vi "Remove - Update Poly Set Map.vi"(8 "error in (no error)":errorcluster, 10 "Data Type to Remove":string[](array[string]), 11 "Poly Set Map in in":T1) -> (0 "error out":errorcluster, 1 "Data Type Library Path":path, 2 "Data Type Directory":path, 3 "Poly Set Map out":T1)   [LabVIEW 2020]
uses:
  _td_map_PolyInstanceInfo.ctl
  _td_cluster_InstanceInfo.ctl
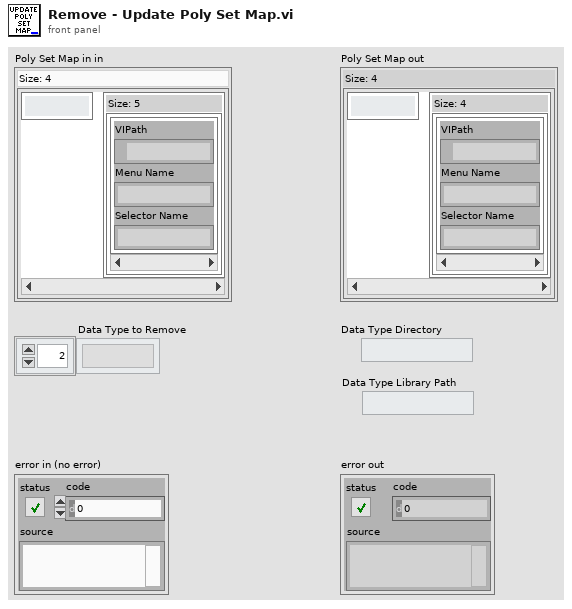
[diagram p1: front panel]
types:
  T1 = typedef "_td_map_PolyInstanceInfo.ctl" = map{string, set{T2}}
  T2 = typedef "_td_cluster_InstanceInfo.ctl" = cluster{"VIPath":path, "Menu Name":string, "Selector Name":string}
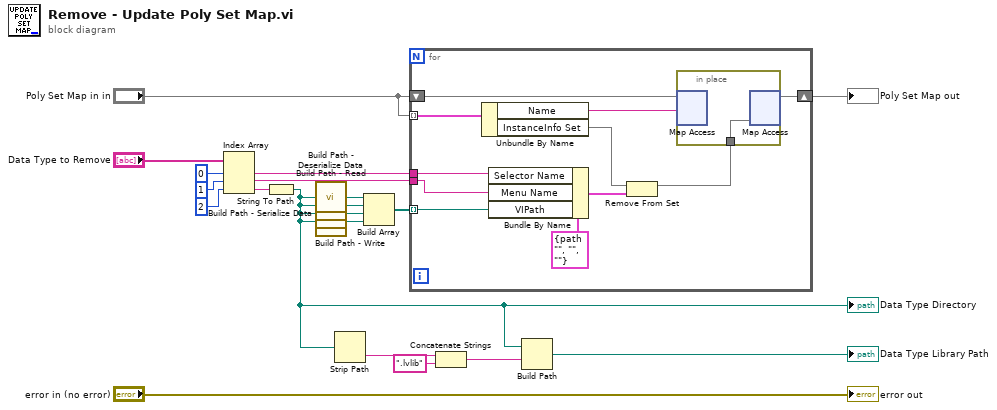
[diagram p0: block diagram]
diagram:
  n1 = Index Array(array="Data Type to Remove", index #1=0 ("index"), index #2=1 ("index"), index #3=2 ("index")) -> (element #1=w13:string, element #2=w12:string, element #3=w9:string)
  n2 = String To Path(string=w9) -> (path=w5:path)
  "Data Type Directory" <- w5
  n3 = call "Build Path - Deserialize Data.vi"("Directory"=w5) -> ("Path to Deserialize Data.vi"=w15:path)
  n4 = call "Build Path - Read.vi"("Directory"=w5) -> ("Path to Read.vi"=w16:path)
  n5 = call "Build Path - Serialize Data.vi"("Directory"=w5) -> ("Path to Serialize Data.vi"=w17:path)
  n6 = call "Build Path - Write.vi"("Directory"=w5) -> ("Path to Write.vi"=w18:path)
  n7 = Strip Path(path=w5) -> (name=w4:string)  [unwired: 1 out]
  n8 = Build Array(w15, w16, w17, w18) -> (w19:path[])
  n9 = for {
    tunnel: "Poly Set Map in in" -> [w31] mode=indexing
    tunnel: w12 -> [w30]
    tunnel: w13 -> [w29]
    shift-right: [w23] -> w20
    shift-left: "Poly Set Map in in" -> [w26]
    tunnel: w19 -> [w21] mode=indexing
    n10 = Unbundle By Name(w31) -> ("Name"=w24:string, "InstanceInfo Set"=w27:set{T2})
    n11 = Bundle By Name(cluster=T2 {"VIPath"=path "", "Menu Name"="", "Selector Name"=""} ("InstanceInfo"), "Selector Name"=w29, "Menu Name"=w30, "VIPath"=w21) -> (w22:T2)
    n12 = Remove From Set(10:w22, 11:w27) -> (3:w25:set{T2})  [unwired: 1 out]
    n13 = in-place {
      in-place-border: w25 -> [w32]
      n14 = in-place-map #1(w26, w24) -> ()  [unwired: 1 in, 2 out]
      n15 = in-place-map #1(w32) -> (w23:T1)  [unwired: 1 in, 2 out]
    }
  }
  "Poly Set Map out" <- w20
  n16 = Concatenate Strings(w4, ".lvlib" ("string")) -> (w2:string)
  n17 = Build Path(base path=w5, name or relative path=w2) -> (appended path=→"Data Type Library Path":path)
  "error out" <- "error in (no error)"
